vi "Process.vi"(8 "error in (no error)":errorcluster, 9 "Panel":refnum<class "Panel Controller Interface.lvclass">, 10 "Console Reply.lvclass":refnum<class "Console Reply.lvclass">, 11 "Add Control In Panel_Msg":refnum<class "Add Control_Behavior.lvclass">) -> (0 "error out":errorcluster, 3 "Add Control In Panel_Msg":refnum<class "Add Control_Behavior.lvclass">)   [LabVIEW 2015, in "Add Control_Behavior.lvclass"]
uses:
  Add Control_Behavior.lvclass
  _Depences/Panel API/Console Reply/Console Reply/Console Reply.lvclass
  _Depences/Panel API/Panel Control_Interface/Panel_interface/Panel Controller Interface.lvclass
  Panel Control_Ref/Panel Controller.lvclass
  _Depences/Panel API/Console Reply/Console Reply/Console Reply.lvclass/Console Reply.ctl
  Add Control_Behavior.lvclass/Add Control_Behavior.ctl
  GUI/GUI Controls/GUI Control/GUI Control.lvclass
  Panel GUI Manager/Panel GUI Manager.lvclass
  GUI/GUI Builder Director/GUI Control Builder Director.lvclass
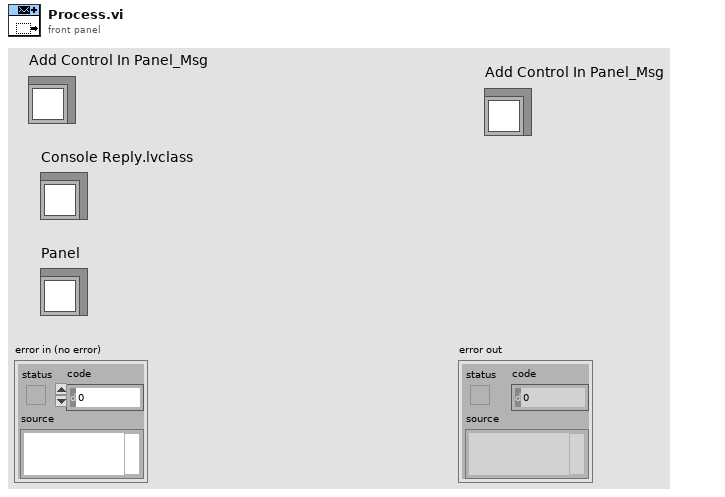
[diagram p1: front panel]
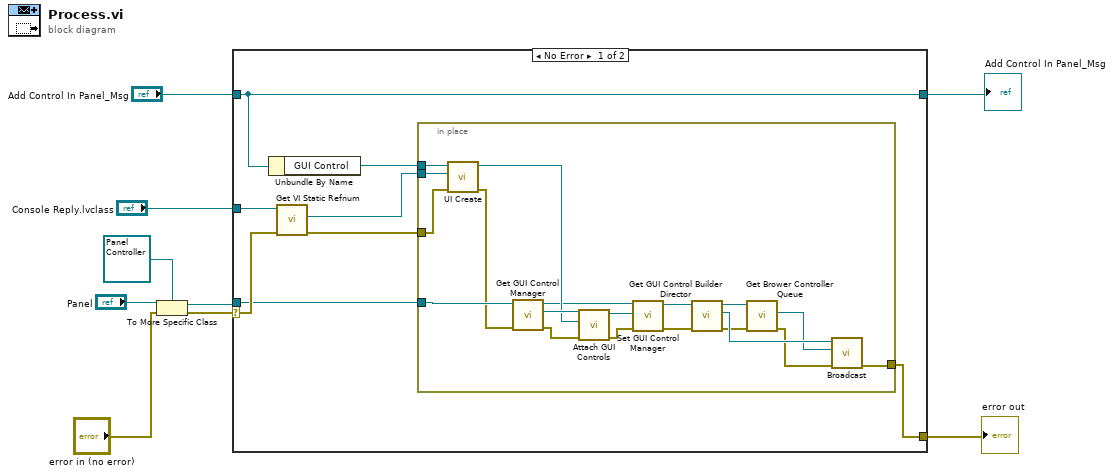
[diagram p0: block diagram]
diagram:
  n1 = To More Specific Class(target class=refnum<class "Panel Controller.lvclass"> refnum ("Panel Control_Ref"), reference="Panel", error in="error in (no error)") -> (specific class reference=w1:refnum<class "Panel Controller.lvclass">, error out=w2:errorcluster)
  n2 = case shown="No Error" w2 {
    selector: w2 -> [w16 w38]
    tunnel: [w10 w38] -> w9
    tunnel: [w11 w37] -> w7
    tunnel: "Add Control In Panel_Msg" -> [w11 w37]
    tunnel: "Console Reply.lvclass" -> [w17 _]
    tunnel: w1 -> [w12 _]
    frame No Error {
      n3 = Unbundle By Name(w11) -> ("GUI Control"=w15:refnum<class "GUI Control.lvclass">)
      n4 = call "Get VI Static Refnum.vi"("error in (no error)"=w16, "Console Reply in"=w17) -> ("error out"=w13:errorcluster, "VI Static Refnum"=w14:refnum<vi>)  [unwired: 7 in, 1 out]
      n5 = in-place {
        in-place-border: w15 -> [w36]
        in-place-border: w14 -> [w35]
        in-place-border: w13 -> [w34]
        in-place-border: w12 -> [w33]
        in-place-border: [w18] -> w10
        n6 = call-dynamic "UI Create.vi"("error in (no error)"=w34, "VI Refnum"=w35, "GUI Control in"=w36) -> ("error out"=w29:errorcluster, "GUI Control out"=w31:refnum<class "GUI Control.lvclass">)  [unwired: 7 in]
        n7 = call "Get GUI Control Manager.vi"("error in (no error)"=w29, "Panel Control_Ref in"=w33) -> ("error out"=w30:errorcluster, "Panel GUI Manager.lvclass"=w32:refnum<class "Panel GUI Manager.lvclass">, "Panel Control_Ref out"=w28:refnum<class "Panel Controller.lvclass">)  [unwired: 7 in]
        n8 = call "Attach GUI Controls.vi"("error in (no error)"=w30, "GUI Control.lvclass"=w31, "Panel GUI Manager in"=w32) -> ("error out"=w26:errorcluster, "Panel GUI Manager out"=w27:refnum<class "Panel GUI Manager.lvclass">)  [unwired: 7 in]
        n9 = call "Set GUI Control Manager.vi"("error in (no error)"=w26, "Panel GUI Manager.lvclass"=w27, "Panel Control_Ref in"=w28) -> ("error out"=w24:errorcluster, "Panel Control_Ref out"=w25:refnum<class "Panel Controller.lvclass">)  [unwired: 7 in]
        n10 = call "Get GUI Control Builder Director.vi"("error in (no error)"=w24, "Panel Control_Ref in"=w25) -> ("error out"=w20:errorcluster, "GUI Control Builder Director.lvclass"=w22:refnum<class "GUI Control Builder Director.lvclass">, "Panel Control_Ref out"=w23:refnum<class "Panel Controller.lvclass">)  [unwired: 7 in]
        n11 = call "Get Brower Controller Queue.vi"("error in (no error)"=w20, "Panel Control_Ref in"=w23) -> ("error out"=w19:errorcluster, "Brower Controller_Q"=w21:refnum<class "Message Enqueuer.lvclass">)  [unwired: 7 in, 1 out]
        n12 = call "Broadcast.vi"("error in (no error)"=w19, "Brower Controller_Q"=w21, "GUI Control Builder Director in"=w22) -> ("error out"=w18:errorcluster)  [unwired: 7 in, 1 out]
      }
    }
    frame Error {
    }
  }
  "error out" <- w9
  "Add Control In Panel_Msg" <- w7
